vi "Gif Picture Grab.vi"(6 "picture background":picture, 7 "images":T1[](array[typedef]), 8 "error in (no error)":errorcluster, 11 "Pop-Up.lvlib:Gif Parent.lvclass":refnum<class "Gif Parent.lvclass">) -> (0 "error out":errorcluster, 2 "1st picture":picture, 3 "Pop-Up.lvlib:Gif Parent.lvclass out":refnum<class "Gif Parent.lvclass">)   [LabVIEW 2020, in "Pop-Up.lvlib" / "Gif Parent.lvclass"]
doc: "read the information for the custom image \n\n<b>Code Developed By:</b>\nTechnology Service Corporation\n1983 S Liberty Drive\nBloomington, IN 47403\nPhone: 812 558-7100\nwww.tsc.com/atcs"
uses:
  Gif Parent.lvclass
  <vilib>/picture/picture.llb/imagedata.ctl
  Gif Parent.lvclass/Gif Parent.ctl
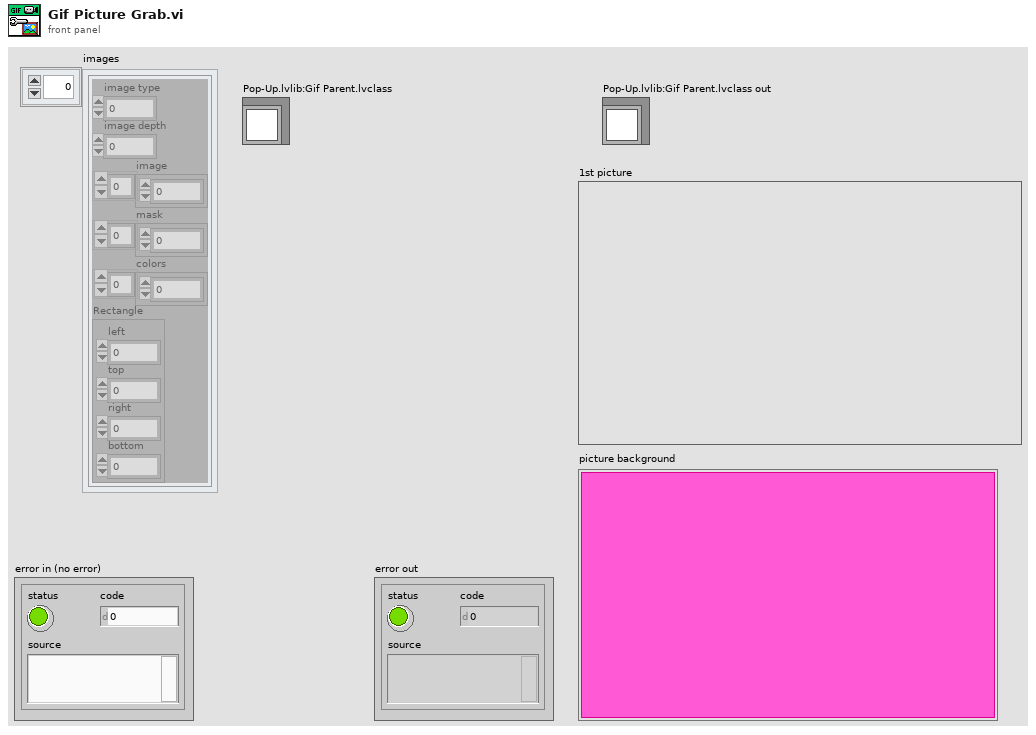
[diagram p1: front panel]
types:
  T1 = typedef "imagedata.ctl" = cluster{"image type":i32, "image depth":i32, "image":u8[], "mask":u8[], "colors":u32[], "Rectangle":cluster{"left":i16, "top":i16, "right":i16, "bottom":i16}}
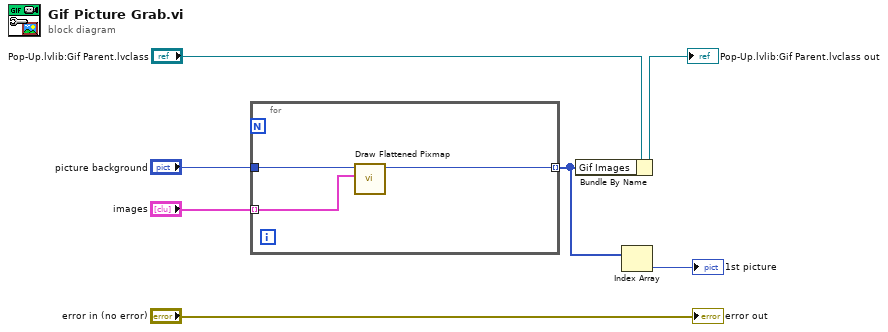
[diagram p0: block diagram]
diagram:
  n1 = for {
    tunnel: "images" -> [w8] mode=indexing
    tunnel: "picture background" -> [w9]
    tunnel: [w10] -> w2 mode=indexing
    n2 = call <vilib>:"Draw Flattened Pixmap.vi"("image data"=w8, "picture"=w9) -> ("new picture"=w10:picture)  [unwired: 7 in]
  }
  n3 = Bundle By Name(cluster="Pop-Up.lvlib:Gif Parent.lvclass", "Gif Images"=w2) -> (→"Pop-Up.lvlib:Gif Parent.lvclass out":refnum<class "Gif Parent.lvclass">)
  n4 = Index Array(array=w2) -> (element=→"1st picture":picture)  [unwired: 1 in]
  "error out" <- "error in (no error)"
